vi "Get Object Items by Item Names.vi"(7 "Item Names":string[](array[string]), 8 "error in (no error)":errorcluster, 10 "Object Offset":i32, 11 "JSON":string) -> (0 "error out":errorcluster, 1 "<JSON>":string[](array[string]) caption="Found Items<JSON>", 2 "Names":string[](array[string]))   [LabVIEW 2013, in "JSONtext.lvlib"]
uses:
  JSONtext.lvlib
  support/Unescape JSON string.vi
  support/JSONtext support.lvlib
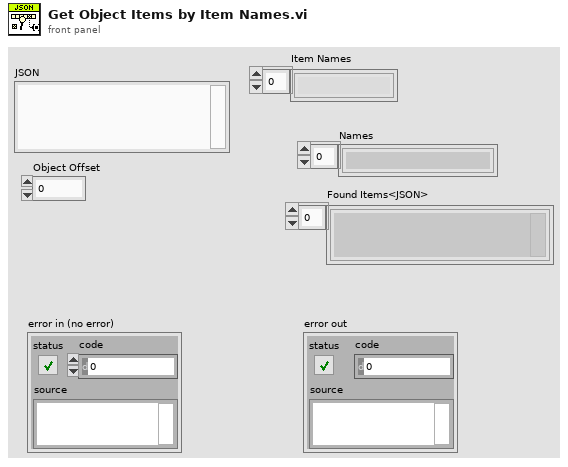
[diagram p1: front panel]
types:
  T1 = typedef "JSONtext.lvlib/Found Items.ctl" = cluster{"Item offset":i32, "Offset past Item":i32, "Name offset":i32, "Offset past Name":i32, "Found":bool, "Empty Object":bool}
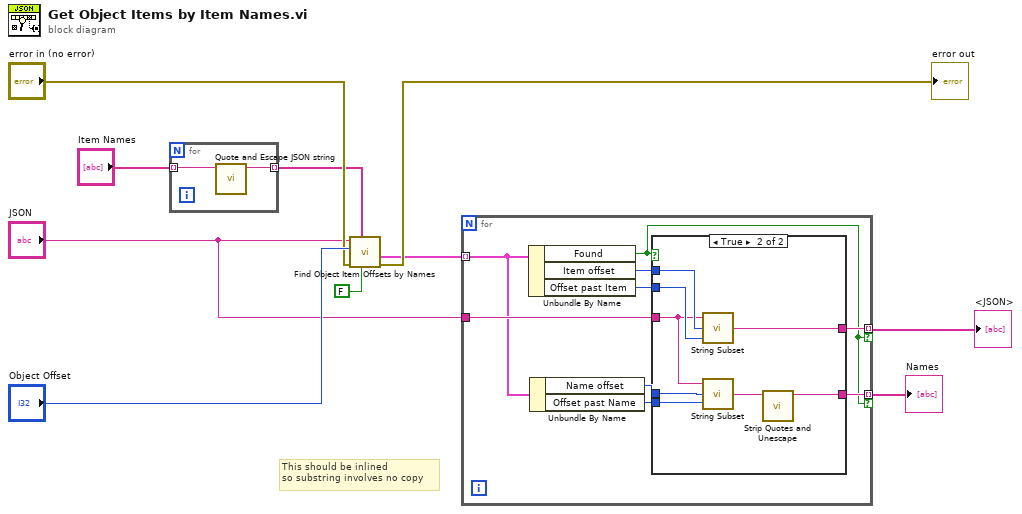
[diagram p0: block diagram]
diagram:
  # "This should be inlined\nso substring involves no copy"
  n1 = for {
    tunnel: "Item Names" -> [w12] mode=indexing
    tunnel: [w11] -> w1 mode=indexing
    n2 = call "Quote and Escape JSON string.vi"("Plain Text"=w12) -> ("<JSON>"=w11:string)  [unwired: 10 in]
  }
  n3 = call "Find Object Item Offsets by Names.vi"("Only return first found"=FALSE, "Item Names <JSON>"=w1, "error in (no error)"="error in (no error)", "Object Offset"="Object Offset", "JSON"="JSON") -> ("error out"=→"error out":errorcluster, "Items"=w5:T1[])  [unwired: 5 in]
  n4 = for {
    tunnel: "JSON" -> [w21]
    tunnel: [w20] -> w6 mode=indexing if=w13
    tunnel: w5 -> [w17] mode=indexing
    tunnel: [w14] -> w4 mode=indexing if=w13
    n5 = Unbundle By Name(w17) -> ("Found"=w13:bool, "Item offset"=w19:i32, "Offset past Item"=w18:i32)
    n6 = Unbundle By Name(w17) -> ("Name offset"=w15:i32, "Offset past Name"=w16:i32)
    n7 = case shown="True" w13 {
      tunnel: w21 -> [_ w26]
      tunnel: [_ w29] -> w20
      tunnel: w19 -> [_ w28]
      tunnel: w18 -> [_ w27]
      tunnel: w16 -> [_ w25]
      tunnel: w15 -> [_ w24]
      tunnel: [_ w22] -> w14
      frame False {
      }
      frame True {
        n8 = call "String Subset.vi"("Offset past End"=w27, "Start offset"=w28, "JSON"=w26) -> ("substring"=w29:string)  [unwired: 2 in]
        n9 = call "String Subset.vi"("Offset past End"=w25, "Start offset"=w24, "JSON"=w26) -> ("substring"=w23:string)  [unwired: 2 in]
        n10 = call "Strip Quotes and Unescape.vi"("String"=w23) -> ("result string"=w22:string)  [unwired: 9 in, 1 out]
      }
    }
  }
  "<JSON>" <- w6
  "Names" <- w4
